vi "Disconnect.vi"(8 "error in (no error)":errorcluster, 9 "Connection Name":string) -> (0 "error out":errorcluster, 2 "isSshConnected":bool, 3 "Return String":string)   [LabVIEW 2022 SP3, in "LabSSH.lvlib"]
doc: "<License>This software is distributed under the BSD 3-Clause License. For the full license please see license.txt or visit www.labvolution.com/license</License>"
uses:
  LabSSH.lvlib
  FGV State..enum.ctl
  <vilib>/Utility/error.llb/Error Cluster From Error Code.vi
  D:/project/tvtEye/guard_tvt/tools/LabSSH Library/References/LabSSH.dll
  References/LabSSH.dll
  <vilib>/ErrorRing/Error Ring.xnode
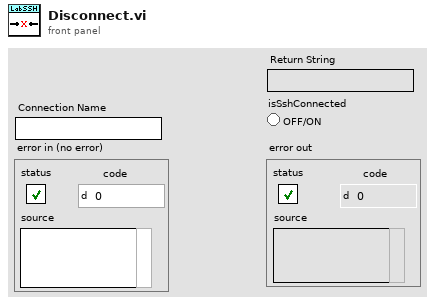
[diagram p1: front panel]
types:
  T1 = typedef "LabSSH.lvlib/FGV State..enum.ctl" = enum16{"GET", "SET"}
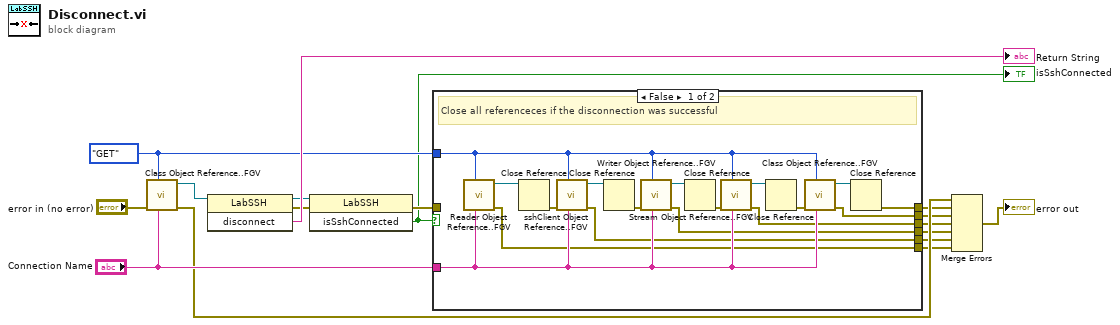
[diagram p0: block diagram]
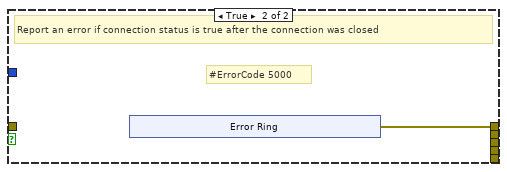
[diagram p2: hidden frame]
diagram:
  w13 = FGV_State..enum."GET" ("FGV State")
  n1 = call "Class Object Reference..FGV.vi"("Connection Name"="Connection Name", "FGV State (GET)"=w13, "error in (no error)"="error in (no error)") -> ("error out"=w8:errorcluster, "LabSSH ref out"=w15:refnum<k24>)  [unwired: 7 in]
  n2 = invoke class="LabSSH" method="disconnect"(reference=w15) -> (reference out=w11:refnum<k24>, error out=w14:errorcluster, "disconnect"=→"Return String":string)  [unwired: 2 in]
  n3 = invoke class="LabSSH" method="isSshConnected"(reference=w11, error in=w14) -> (error out=w12:errorcluster, "isSshConnected"=w10:bool)  [unwired: 1 in, 1 out]
  "isSshConnected" <- w10
  n4 = case shown="False" w10 {
    tunnel: w13 -> [w34 _]
    tunnel: [w33 w35] -> w6
    tunnel: w12 -> [_ _]
    tunnel: "Connection Name" -> [w26 _]
    tunnel: [w22 _] -> w5
    tunnel: [w21 _] -> w4
    tunnel: [w20 _] -> w3
    tunnel: [w19 _] -> w2
    tunnel: [w18 _] -> w1
    frame False {
      # "Close all referenceces if the disconnection was successful"
      n5 = call "Reader Object Reference..FGV.vi"("Connection Name"=w26, "FGV State (GET)"=w34) -> ("error out"=w18:errorcluster, "Reader ref out"=w29:refnum<k24>)  [unwired: 8 in]
      n6 = Close Reference(reference=w29) -> (error out=w27:errorcluster)  [unwired: 1 in]
      n7 = call "sshClient Object Reference..FGV.vi"("Connection Name"=w26, "FGV State (GET)"=w34, "error in (no error)"=w27) -> ("error out"=w19:errorcluster, "sshClient ref out"=w28:refnum<k24>)  [unwired: 7 in]
      n8 = Close Reference(reference=w28) -> (error out=w25:errorcluster)  [unwired: 1 in]
      n9 = call "Writer Object Reference..FGV.vi"("Connection Name"=w26, "FGV State (GET)"=w34, "error in (no error)"=w25) -> ("error out"=w20:errorcluster, "Writer ref out"=w30:refnum<k24>)  [unwired: 7 in]
      n10 = Close Reference(reference=w30) -> (error out=w24:errorcluster)  [unwired: 1 in]
      n11 = call "Stream Object Reference..FGV.vi"("Connection Name"=w26, "FGV State (GET)"=w34, "error in (no error)"=w24) -> ("error out"=w21:errorcluster, "Stream ref out"=w31:refnum<k24>)  [unwired: 7 in]
      n12 = Close Reference(reference=w31) -> (error out=w23:errorcluster)  [unwired: 1 in]
      n13 = call "Class Object Reference..FGV.vi"("Connection Name"=w26, "FGV State (GET)"=w34, "error in (no error)"=w23) -> ("error out"=w22:errorcluster, "LabSSH ref out"=w32:refnum<k24>)  [unwired: 7 in]
      n14 = Close Reference(reference=w32) -> (error out=w33:errorcluster)  [unwired: 1 in]
    }
    frame True {
      # "#ErrorCode 5000"
      # "Report an error if connection status is true after the connection was closed"
      n15 = xnode "Error Ring"() -> ("error out"=w35:errorcluster)
    }
  }
  n16 = Merge Errors(w8, w6, w5, w4, w3, w2, w1) -> (→"error out":errorcluster)
